vi "G#Debugger_Close.vi"(0 "refs":T1, 5 "error in (no error)":errorcluster) -> (19 "error out":errorcluster)   [LabVIEW 2017, in "G#Debugger.lvlib"]
uses:
  G#Debugger.lvlib
  G#Debugger_Refs.ctl
  G#Object/utils/G#Object_ClassInfoType.ctl
  G#Object/G#Object.lvclass
  G#Object/utils/G#Object_ObjectInfoType.ctl
  G#Object/utils/G#Object_CreateMethod.ctl
  G#Debugger_SubPanelInfo.ctl
  G#Object/utils/G#Object_ClassHierarchy.ctl
  G#RemoteProxy/G#RemoteProxy.lvclass
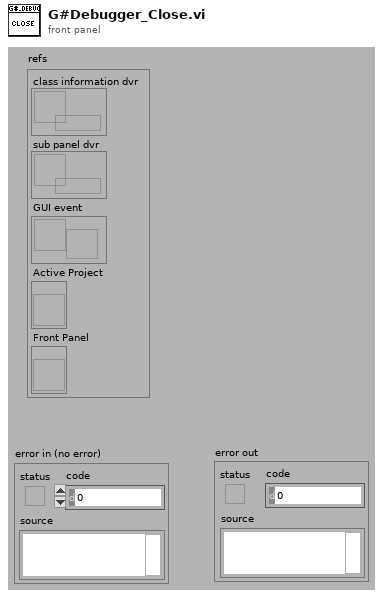
[diagram p1: front panel]
types:
  T1 = typedef "G#Debugger.lvlib/G#Debugger_Refs.ctl" = cluster{"class information dvr":refnum<data-value>, "sub panel dvr":refnum<data-value>, "GUI event":refnum<user-event>, "Active Project":refnum<vi>, "Front Panel":refnum<vi>}
  T2 = typedef "G#Debugger.lvlib/G#Debugger_SubPanelInfo.ctl" = cluster{"Ref":refnum<class "G#Object.lvclass">, "class hierarchy":T3[], "class attributes":path[], "object attributes":path[], "inheritance index":i32, "is class attributes":bool, "vi reference":refnum<vi>}
  T3 = typedef "G#Object.lvclass/G#Object_ClassHierarchy.ctl" = cluster{"ClassName":string, "FullClassName":string, "ClassPath":path, "IsLeaf":bool}
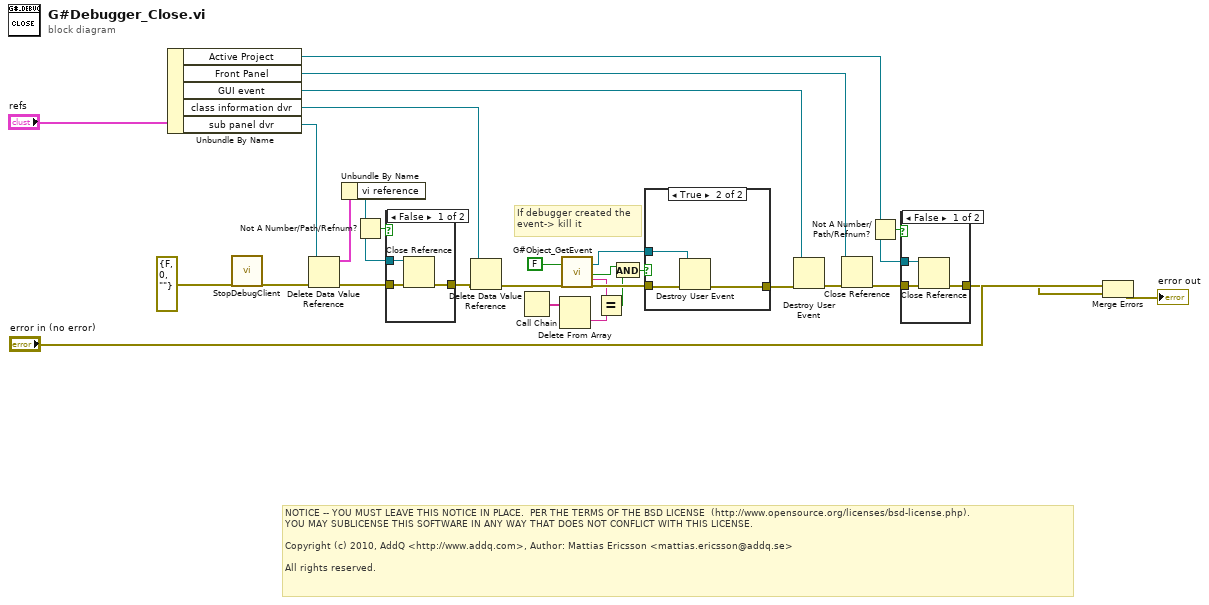
[diagram p0: block diagram]
diagram:
  # "If debugger created the\nevent-> kill it"
  # "NOTICE -- YOU MUST LEAVE THIS NOTICE IN PLACE.  PER THE TERMS OF THE BSD LICENSE  (http://www.opensource.org/licenses/bsd-license.php).\nYOU MAY SUBLICENSE THIS SOFTWARE IN ANY WAY THAT DOES NOT CONFLICT WITH THIS LICENSE.\n\nCopyright (c) 2010, AddQ <http://www.addq.com>, Author: Mattias Ericsson <mattias.ericsson@addq.se>\n\nAll rights reserved."
  n1 = Unbundle By Name("refs") -> ("Active Project"=w12:refnum<vi>, "Front Panel"=w1:refnum<vi>, "GUI event"=w20:refnum<user-event>, "class information dvr"=w23:refnum<data-value>, "sub panel dvr"=w24:refnum<data-value>)
  n2 = call "StopDebugClient.vi"("error in (no error)"=errorcluster {"status"=FALSE, "code"=0, "source"=""}) -> ("error out"=w4:errorcluster)  [unwired: 18 in]
  n3 = Delete Data Value Reference(data value reference=w24, error in=w4) -> (data value=w29:T2, error out=w28:errorcluster)
  n4 = Unbundle By Name(w29) -> ("vi reference"=w25:refnum<vi>)
  n5 = Not A Number/Path/Refnum?(number/path/refnum=w25) -> (NaN/Path/Refnum?=w27:bool)
  n6 = case shown="False" w27 {
    tunnel: w28 -> [w33 w34]
    tunnel: [w32 w34] -> w26
    tunnel: w25 -> [w31 _]
    frame False {
      n7 = Close Reference(reference=w31, error in (no error)=w33) -> (error out=w32:errorcluster)
    }
    frame True {
    }
  }
  n8 = Delete Data Value Reference(data value reference=w23, error in=w26) -> (error out=w19:errorcluster)  [unwired: 1 out]
  n9 = Call Chain() -> (call chain=w10:string[])
  n10 = Delete From Array(array=w10) -> (deleted portion=w9:string)  [unwired: 2 in, 1 out]
  n11 = call "G#Object_GetEvent.vi"("create if needed (T)"=FALSE ("create if needed"), "error in (no error)"=w19) -> ("G# event"=w15:refnum<user-event>, "valid"=w7:bool, "event owner"=w8:string, "error out"=w17:errorcluster)  [unwired: 13 in, 1 out]
  n12 = Equal?(x=w8, y=w9) -> (x = y?=w6:bool)
  n13 = And(x=w7, y=w6) -> (x .and. y?=w16:bool)
  n14 = case shown="True" w16 {
    tunnel: w17 -> [w35 w38]
    tunnel: w15 -> [_ w37]
    tunnel: [w35 w36] -> w14
    frame False {
    }
    frame True {
      n15 = Destroy User Event(user event=w37, error in=w38) -> (error out=w36:errorcluster)
    }
  }
  n16 = Destroy User Event(user event=w20, error in=w14) -> (error out=w3:errorcluster)
  n17 = Close Reference(reference=w1, error in (no error)=w3) -> (error out=w2:errorcluster)
  n18 = Not A Number/Path/Refnum?(number/path/refnum=w12) -> (NaN/Path/Refnum?=w13:bool)
  n19 = case shown="False" w13 {
    tunnel: w2 -> [w41 w42]
    tunnel: [w40 w42] -> w11
    tunnel: w12 -> [w39 _]
    frame False {
      n20 = Close Reference(reference=w39, error in (no error)=w41) -> (error out=w40:errorcluster)
    }
    frame True {
    }
  }
  n21 = Merge Errors("error in (no error)", w11) -> (→"error out":errorcluster)
